vi "Pre Launch Init.vi"(11 "ArduinoTranslationStage in":refnum<class "ArduinoTranslationStage.lvclass">) -> (0 "error out":errorcluster, 3 "ArduinoTranslationStage out":refnum<class "ArduinoTranslationStage.lvclass">)   [LabVIEW 2023]
doc: "(<B>Filename</B>: Actor Framework.lvlib:Actor.lvclass:Pre Launch Init.vi)\n\nDefines behavior that occurs after the Launch Nested Actor method is invoked but before the actor's Actor Core method begins running.\n\nBy default, this method does nothing. A descendant class may override it to define behavior."
uses:
  ArduinoTranslationStage.lvclass
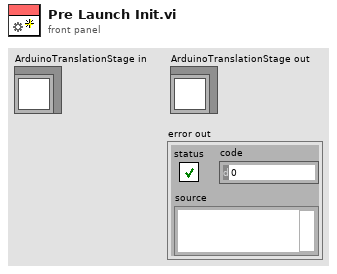
[diagram p1: front panel]
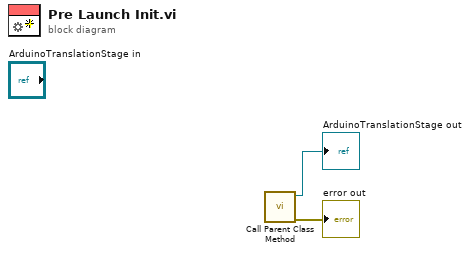
[diagram p0: block diagram]
diagram:
  n1 = call-parent "Call Parent Class Method"() -> ("error out"=→"error out":errorcluster, "Actor out"=→"ArduinoTranslationStage out":refnum<class "ArduinoTranslationStage.lvclass">, "Actor in"=w2:refnum<class "ArduinoTranslationStage.lvclass">)  [unwired: 9 in]
